vi "Recall Channel State.vi"(8 "error in (no error)":errorcluster, 10 "Memory Register (0: A)":u16(ring) items=["A", "B", "C", "D"], 11 "VISA resource name":refnum<visa-resource-name>) -> (0 "error out":errorcluster, 3 "VISA resource name out":refnum<visa-resource-name>)   [LabVIEW 2018, in "Agilent ENA Series.lvlib"]
doc: "Recalls the instrument state for an individual channel from the specified register as the setting of the active channel.\n\nNotes:\nIt is possible to recall the register from a different channel where it was saved."
uses:
  Agilent ENA Series.lvlib
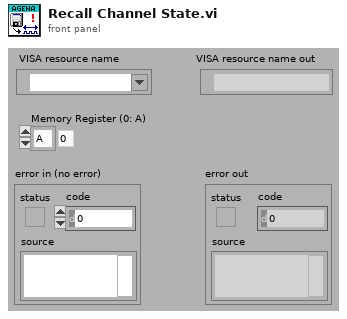
[diagram p1: front panel]
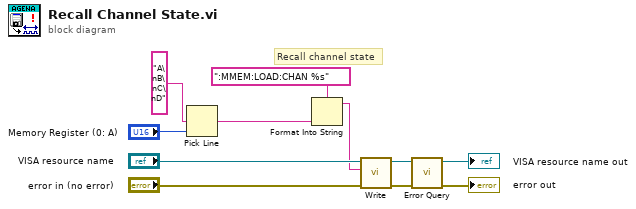
[diagram p0: block diagram]
diagram:
  # "Recall channel state"
  n1 = Pick Line(multi-line string="A\nB\nC\nD", line index="Memory Register (0: A)") -> (output string=w5:string)  [unwired: 1 in]
  n2 = Format Into String(format string=":MMEM:LOAD:CHAN %s", w5) -> (resulting string=w8:string)  [unwired: 2 in, 1 out]
  n3 = call "Write.vi"("error in (no error)"="error in (no error)", "String ()"=w8, "VISA resource name"="VISA resource name") -> ("error out"=w3:errorcluster, "VISA resource name out"=w4:refnum<visa-resource-name>)  [unwired: 6 in, 1 out]
  n4 = call "Error Query.vi"("error in (no error)"=w3, "VISA resource name"=w4) -> ("error out"=→"error out":errorcluster, "VISA resource name out"=→"VISA resource name out":refnum<visa-resource-name>)  [unwired: 6 in, 2 out]
